vi "GetStatus EC.vi"(8 "error in (no error)":errorcluster, 11 "TCP Network Connection in":refnum<k5>) -> (0 "error out":errorcluster, 3 "Status":T1)   [LabVIEW 2011]
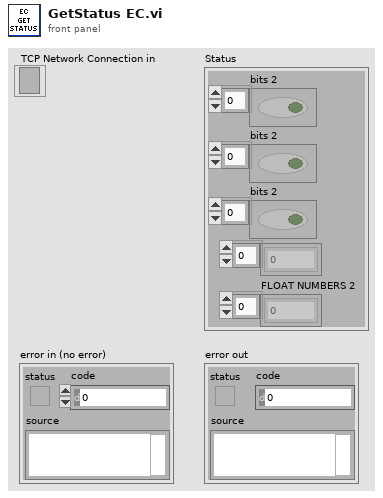
[diagram p1: front panel]
types:
  T1 = cluster{"bits 2":bool[], "bits 2":bool[], "bits 2":bool[], i32[], "FLOAT NUMBERS 2":sgl[]}
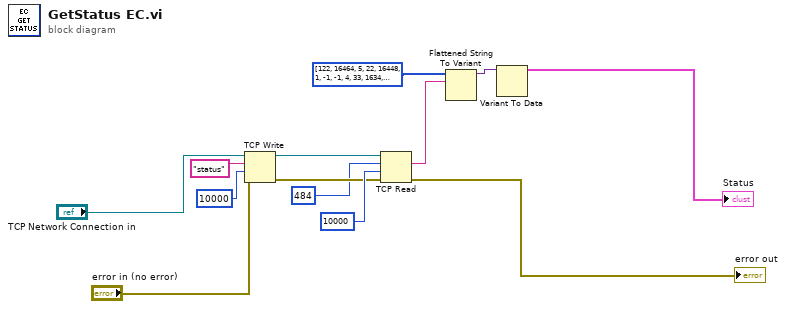
[diagram p0: block diagram]
diagram:
  n1 = TCP Write(connection ID="TCP Network Connection in", data in="status", error in (no error)="error in (no error)", 9:10000 ("timeout ms (25000)")) -> (connection ID out=w8:refnum<k5>, error out=w7:errorcluster)  [unwired: 1 out]
  n2 = TCP Read(connection ID=w8, bytes to read=484 ("length"), error in (no error)=w7, 9:10000 ("ms timeout (10000)")) -> (data out=w10:string, error out=→"error out":errorcluster)  [unwired: 1 in, 1 out]
  n3 = Flattened String To Variant(6:w10, 7:i16[] [122, 16464, 5, 22, 16448, 1, -1, -1, 4, 33, 1634, 26996, 29472, 12800, 22, 16448, 1, -1, -1, 4, 33, 1634, 26996, 29472, 12800, 22, 16448, 1, -1, -1, 4, 33, 1634, 26996, 29472, 12800, 14, 64, 1, -1, -1, 4, 3, 30, 16448, 1, -1, -1, 4, 9, 3910, 19535, 16724, 8270, 21837, 16965, 21075, 8242, 1092, 16724, 16640] ("type string")) -> (3:w9:variant)  [unwired: 1 in, 1 out]
  n4 = Variant To Data(Variant=w9) -> (data=→"Status":T1)  [unwired: 2 in, 1 out]
